vi "iHR550 Set Values v10.6.2.vi"(0 "Refnum out":refnum<k7>, 1 "Entrance Mirror":u16(ring)=2 caption="Target Position\nEntrance Mirror" items=["Front"=2, "Side"=3], 3 "Target\nSide Entrance":dbl, 5 "iHR Settings":T1={"iHR550 Set Exit Mirror"=2, "iHR550 Set Side Exit"=0.0, "iHR550 Set Front Entrance"=0.0, "iHR550 Set Wavelength"=897.9988, "iHR550 Set Grating"=0, "iHR550 Set Grating Switch"=FALSE, "iHR550 Set Wavelength Switch"=FALSE, "iHR550 Set Mirror Switch"=FALSE, "iHR550 Set Slits Switch"=FALSE} {"iHR550 Set Wavelength" min=0.0 max=1500.0 step=1.0; "iHR550 Set Side Exit" min=0.0 max=2000.0 step=1.0; "iHR550 Set Exit Mirror" items=["Front"=2, "Side"=3]}, 9 "Mono Calibration":path, 11 "error in (no error)":errorcluster, 13 "Target\nFront Exit":dbl) -> (15 "error out":errorcluster)   [LabVIEW 2010]
uses:
  TypeDefs/iHR Settings.ctl
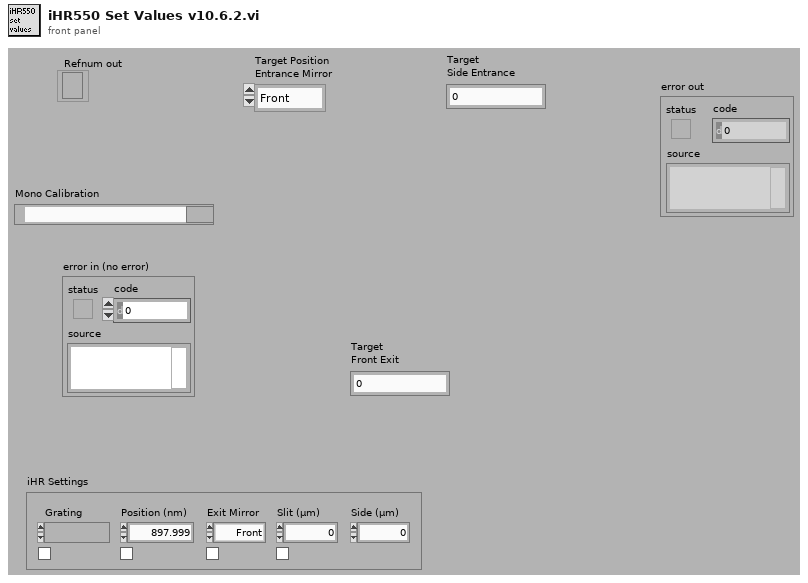
[diagram p1: front panel]
types:
  T1 = typedef "iHR Settings.ctl" = cluster{"iHR550 Set Exit Mirror":u16, "iHR550 Set Side Exit":dbl, "iHR550 Set Front Entrance":dbl, "iHR550 Set Wavelength":dbl, "iHR550 Set Grating":u16, "iHR550 Set Grating Switch":bool, "iHR550 Set Wavelength Switch":bool, "iHR550 Set Mirror Switch":bool, "iHR550 Set Slits Switch":bool}
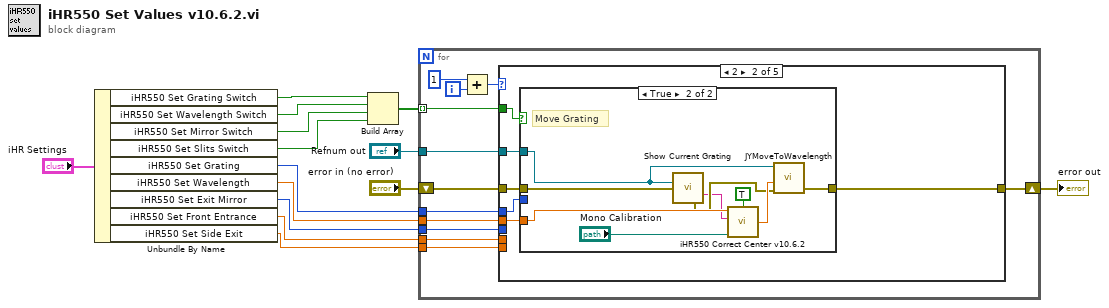
[diagram p0: block diagram]
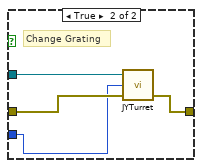
[diagram p3: hidden frame]
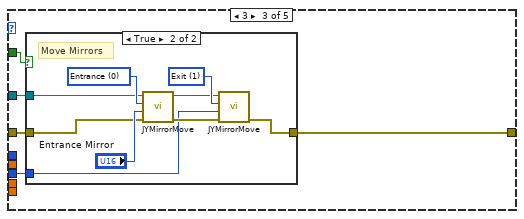
[diagram p5: hidden frame]
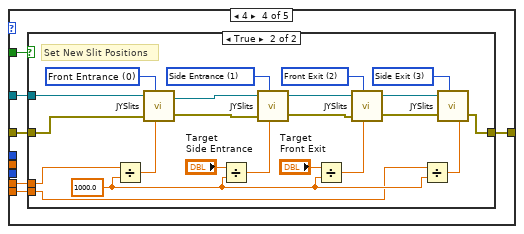
[diagram p7: hidden frame]
diagram:
  n1 = Unbundle By Name("iHR Settings") -> ("iHR550 Set Grating Switch"=w7:bool, "iHR550 Set Wavelength Switch"=w10:bool, "iHR550 Set Mirror Switch"=w9:bool, "iHR550 Set Slits Switch"=w8:bool, "iHR550 Set Grating"=w5:u16, "iHR550 Set Wavelength"=w4:dbl, "iHR550 Set Exit Mirror"=w3:u16, "iHR550 Set Front Entrance"=w2:dbl, "iHR550 Set Side Exit"=w1:dbl)
  n2 = Build Array(w7, w10, w9, w8) -> (w6:bool[])
  n3 = for {
    tunnel: w6 -> [w26] mode=indexing
    tunnel: "Refnum out" -> [w25]
    shift-right: [w24] -> w13
    shift-left: "error in (no error)" -> [w23]
    tunnel: w5 -> [w19]
    tunnel: w4 -> [w18]
    tunnel: w3 -> [w17]
    tunnel: w2 -> [w16]
    tunnel: w1 -> [w15]
    i -> [w22]
    n4 = Add(x=1, y=w22) -> (x+y=w20:i32)
    n5 = case shown="2" w20 {
      tunnel: w26 -> [w31 w39 w54 w73 _]
      tunnel: w25 -> [w30 w40 w55 w70 _]
      tunnel: [w29 w42 w56 w71 w97] -> w24
      tunnel: w23 -> [w28 w41 w57 w72 w97]
      tunnel: w19 -> [w27 w37 _ _ _]
      tunnel: w18 -> [_ w38 _ _ _]
      tunnel: w17 -> [_ _ w53 _ _]
      tunnel: w16 -> [_ _ _ w69 _]
      tunnel: w15 -> [_ _ _ w68 _]
      frame 1 {
        n6 = case shown="False" w31 {
          tunnel: w30 -> [_ w36]
          tunnel: [w32 w35] -> w29
          tunnel: w28 -> [w32 w34]
          tunnel: w27 -> [_ w33]
          frame False {
          }
          frame True {
            # "Change Grating"
            n7 = call "JYTurret.vi"("error in (no error)"=w34, "Grating Index"=w33, "JYMONOLib.IJYMonoReqd"=w36) -> ("error out"=w35:errorcluster)  [unwired: 2 out]
          }
        }
      }
      frame 2 {
        n8 = case shown="True" w39 {
          tunnel: w40 -> [_ w46]
          tunnel: w41 -> [w43 w48]
          tunnel: [w43 w52] -> w42
          tunnel: w38 -> [_ w51]
          tunnel: w37 -> [_ _]
          frame False {
          }
          frame True {
            # "Move Grating"
            n9 = call "Show Current Grating.vi"("Refnum in"=w46, "error in (no error)"=w48) -> ("Current Description"=w45:string, "error out"=w47:errorcluster)  [unwired: 5 in, 7 out]
            n10 = call "iHR550 Correct Center v10.6.2.vi"("Calibration File"="Mono Calibration", "Set?"=TRUE, "Description"=w45, "Position In (nm)"=w51) -> ("Position Out (nm)"=w49:dbl)
            n11 = call "JYMoveToWavelength.vi"("error in (no error)"=w47, "Target WL"=w49, "RefNum In"=w46) -> ("error out"=w52:errorcluster)  [unwired: 1 in, 2 out]
          }
        }
      }
      frame 3 {
        n12 = case shown="True" w54 {
          tunnel: w57 -> [w58 w63]
          tunnel: [w58 w62] -> w56
          tunnel: w55 -> [_ w60]
          tunnel: w53 -> [_ w61]
          frame False {
          }
          frame True {
            w66 = u16 1 items=["Entrance", "Exit", "Front", "Side"] ("Mirror Number")
            w64 = u16 0 items=["Entrance", "Exit", "Front", "Side"] ("Mirror Number")
            # "Move Mirrors"
            n13 = call "JYMirrorMove.vi"("error in (no error)"=w63, "Mirror Position"="Entrance Mirror", "Mirror Number"=w64, "RefNum In"=w60) -> ("error out"=w67:errorcluster, "MonoRefNum Out"=w59:refnum<k7>)  [unwired: 6 in]
            n14 = call "JYMirrorMove.vi"("error in (no error)"=w67, "Mirror Position"=w61, "Mirror Number"=w66, "RefNum In"=w59) -> ("error out"=w62:errorcluster)  [unwired: 6 in, 1 out]
          }
        }
      }
      frame 4 {
        n15 = case shown="True" w73 {
          tunnel: w72 -> [w74 w86]
          tunnel: [w74 w84] -> w71
          tunnel: w70 -> [_ w85]
          tunnel: w69 -> [_ w76]
          tunnel: w68 -> [_ w75]
          frame False {
          }
          frame True {
            w83 = 1000.0 ("y")
            w96 = u16 3 items=["Front Entrance", "Side Entrance", "Front Exit", "Side Exit", "First Intermediate", "Second Intermediate"] ("Slit")
            w95 = u16 2 items=["Front Entrance", "Side Entrance", "Front Exit", "Side Exit", "First Intermediate", "Second Intermediate"] ("Slit")
            w94 = u16 1 items=["Front Entrance", "Side Entrance", "Front Exit", "Side Exit", "First Intermediate", "Second Intermediate"] ("Slit")
            w93 = u16 0 items=["Front Entrance", "Side Entrance", "Front Exit", "Side Exit", "First Intermediate", "Second Intermediate"] ("Slit")
            # "Set New Slit Positions"
            n16 = Divide(x=w76, y=w83) -> (x/y=w80:dbl)
            n17 = call "JYSlits.vi"("JYMONOLib.IJYMonoReqd"=w85, "Slit"=w93, "error in (no error)"=w86, "Slit Width"=w80) -> ("JYMONOLib.IJYMonoReqd 2"=w87:refnum<k7>, "error out"=w90:errorcluster)  [unwired: 1 in]
            n18 = Divide(x="Target\nSide Entrance", y=w83) -> (x/y=w79:dbl)
            n19 = call "JYSlits.vi"("JYMONOLib.IJYMonoReqd"=w87, "Slit"=w94, "error in (no error)"=w90, "Slit Width"=w79) -> ("JYMONOLib.IJYMonoReqd 2"=w88:refnum<k7>, "error out"=w91:errorcluster)  [unwired: 1 in]
            n20 = Divide(x="Target\nFront Exit", y=w83) -> (x/y=w78:dbl)
            n21 = call "JYSlits.vi"("JYMONOLib.IJYMonoReqd"=w88, "Slit"=w95, "error in (no error)"=w91, "Slit Width"=w78) -> ("JYMONOLib.IJYMonoReqd 2"=w89:refnum<k7>, "error out"=w92:errorcluster)  [unwired: 1 in]
            n22 = Divide(x=w75, y=w83) -> (x/y=w77:dbl)
            n23 = call "JYSlits.vi"("JYMONOLib.IJYMonoReqd"=w89, "Slit"=w96, "error in (no error)"=w92, "Slit Width"=w77) -> ("error out"=w84:errorcluster)  [unwired: 1 in, 1 out]
          }
        }
      }
      frame 5, Default {
      }
    }
  }
  "error out" <- w13
